vi "PicoScope2000aSetEts.vi"(7 "ETS Mode":u32(ring)=1 items=["PS2000A_ETS_OFF", "PS2000A_ETS_FAST", "PS2000A_ETS_SLOW"], 8 "error in (no error)":errorcluster, 9 "etsInterleave":i16=40, 10 "etsCycles":i16=200, 11 "handle in":i16) -> (0 "error out":errorcluster, 3 "handle out":i16, 4 "sampleTimePicoseconds":i32=100)   [LabVIEW 2010]
doc: "Calls SetETS"
uses:
  ps2000a.dll
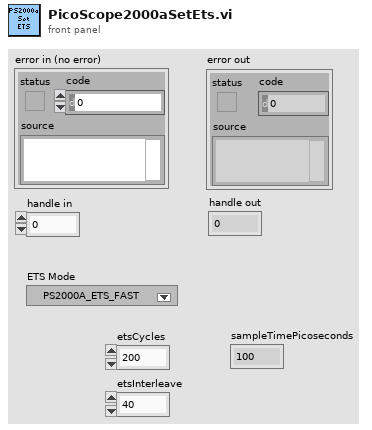
[diagram p1: front panel]
types:
  T1 = cluster{"status":bool, "code":u32, "source":string}
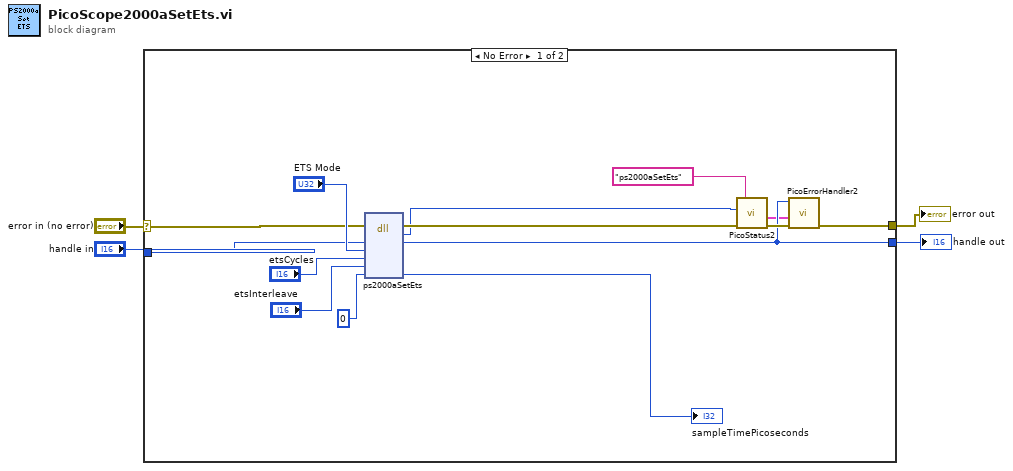
[diagram p0: block diagram]
diagram:
  n1 = case shown="No Error" "error in (no error)" {
    selector: "error in (no error)" -> [w14 w20]
    tunnel: [w17 w20] -> w2
    tunnel: "handle in" -> [w13 w19]
    tunnel: [w9 w19] -> w3
    frame No Error {
      n2 = dll-call lib="ps2000a.dll" fn="ps2000aSetEts" ("ps3000.dll:_ps3000_open_unit@0")(error in=w14, "handle"=w13, "mode"="ETS Mode", "etsCycles"="etsCycles", "etsInterleave"="etsInterleave", "sampleTimePicoseconds"=0) -> (error out=w11:errorcluster, "PICO_STATUS"=w10:u32, "handle"=w9:i16, "sampleTimePicoseconds"=→"sampleTimePicoseconds":i32)  [unwired: 5 in, 1 out]
      n3 = call "PicoStatus2.vi"("PICO source"="ps2000aSetEts" ("source"), "Error in"=w11, "PICO STATUS"=w10) -> ("error out"=w18:errorcluster, "PICO_STATUS out"=w5:T1)  [unwired: 5 in]
      n4 = call "PicoErrorHandler2.vi"("error in (no error)"=w18, "PICO_STATUS in"=w5, "handle In"=w9) -> ("error out"=w17:errorcluster)  [unwired: 8 in]
    }
    frame Error {
    }
  }
  "error out" <- w2
  "handle out" <- w3
